vi "UPH & Target & Clear Zero.vi"(8 "error in (no error)":errorcluster, 11 "Main":T1={"Tite"="", "Base path"=path "", "Table"=[], "Stations"=[], "Shield Array"=[], "UPHs"=[], "VISA"={"VISA"="", "baud rate"=9600, "data bits"=8, "parity"=enum."None", "stop bits"=10, "flow control"=0}, "Path"={"roof"=path "", "Config"=path "", "Png"=path ""}, "Ctr"={"DB Dispaly"=refnum, "Error Table"=refnum, "Display"=refnum, "Login"=refnum, "Exit"=refnum, "FTT_Submit"=refnum}, "Login"={"User"="", "Grade"=""}, "information"={"cause"="", "Type"=enum."Inform", "code"=0, "Suroce"="", "Status"=FALSE}, "Local DB"={"Connstr"="", "Database"={"Constr"={"Driver"="", "Server"="", "User"="", "Pwd"="", "Database"=""}, "conn ref"=refnum, "State"=FALSE}}, "Remote DB"={"Connstr"="", "Database"={"Constr"={"Driver"="", "Server"="", "User"="", "Pwd"="", "Database"=""}, "conn ref"=refnum, "State"=FALSE}}, "FTT TV"="", "ExchangeTime"=0, "NVH"="", "EOL Path"=path ""} {"VISA"."flow control" items=["None", "XON/XOFF", "RTS/CTS", "XON/XOFF & RTS/CTS", "DTR/DSR", "XON/XOFF & DTR/DSR"]; "VISA"."stop bits" items=["1.0"=10, "1.5"=15, "2.0"=20]}) -> (0 "error out":errorcluster)   [LabVIEW 2014]
uses:
  <vilib>/addons/database/Connection.llb/Conn ObjectReference.ctl
  <vilib>/addons/database/NI_Database_API.lvlib
  Type'def/Online_Table.ctl
  Type'def/UPH Config.ctl
  <vilib>/ptbypt/NI_PtbyPt.lvlib
  VISA/Ctr/VISA Ctr.ctl
  Type'def/Main Ctr Ref.ctl
  Type'def/User Login.ctl
  Database/Ctr/Constr.ctl
  Database/Ctr/Conneect State.ctl
  Type'def/MainCtr.ctl
panel:
  in  "Boolean":bool
  out "Previous Event":string
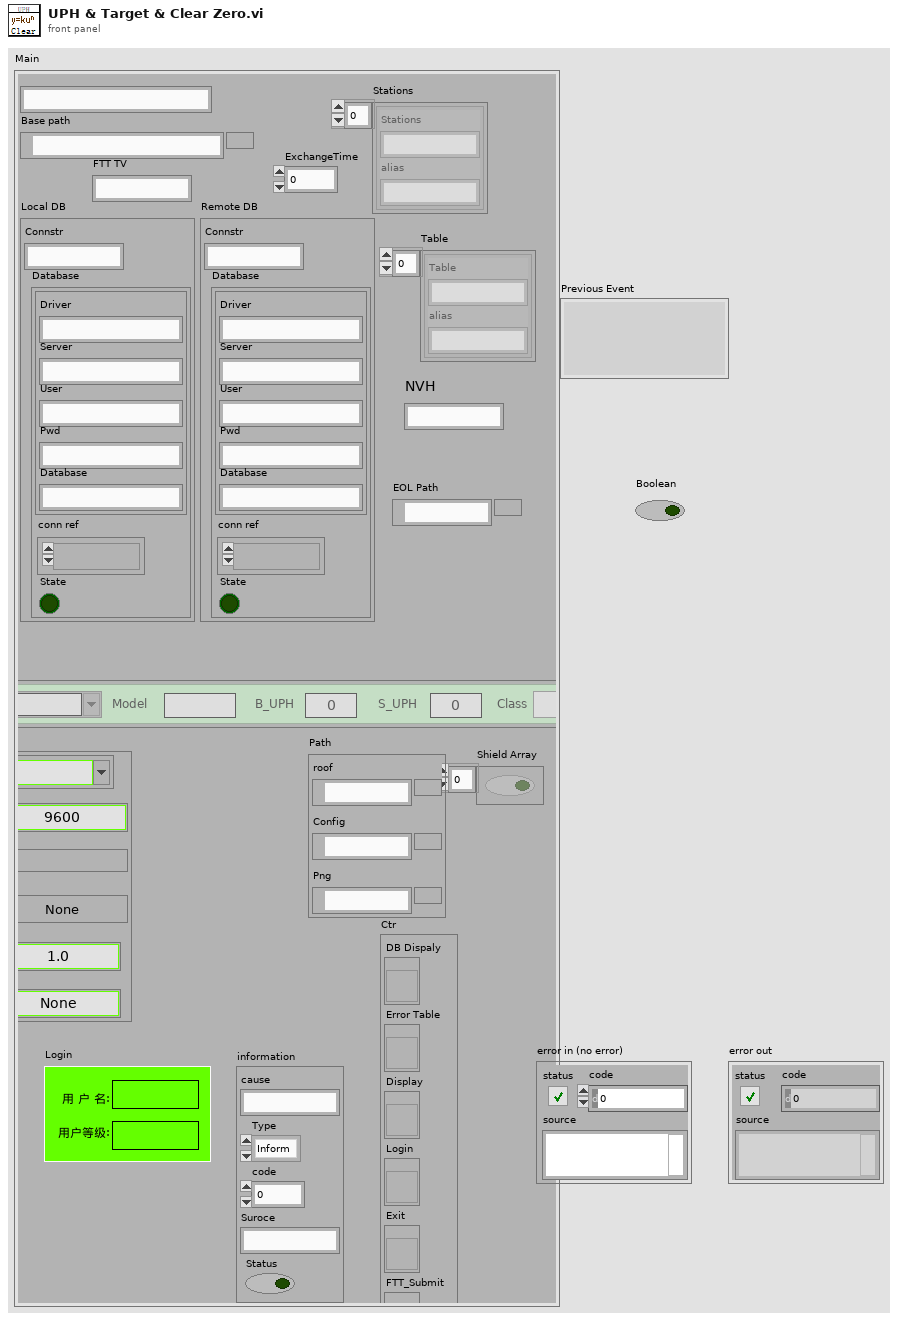
[diagram p1: front panel]
types:
  T1 = typedef "MainCtr.ctl" = cluster{"Tite":string, "Base path":path, "Table":cluster{"Table":string, "alias":string}[], "Stations":cluster{"Stations":string, "alias":string}[], "Shield Array":bool[], "UPHs":T2[], "VISA":T3, "Path":cluster{"roof":path, "Config":path, "Png":path}, "Ctr":T4, "Login":T5, "information":cluster{"cause":string, "Type":enum16{"Inform", "Warning", "Alarm"}, "code":i32, "Suroce":string, "Status":bool}, "Local DB":cluster{"Connstr":string, "Database":T6}, "Remote DB":cluster{"Connstr":string, "Database":T6}, "FTT TV":string, "ExchangeTime":i32, "NVH":string, "EOL Path":path}
  T2 = typedef "UPH Config.ctl" = cluster{"Line_No":string, "Model":string, "B_UPH ":i16, "S_UPH  ":i16, "Class":enum16{"Big", "Small"}}
  T3 = typedef "VISA Ctr.ctl" = cluster{"VISA":refnum<visa-resource-name>, "baud rate":u32, "data bits":u16, "parity":enum16{"None", "Odd", "Even", "Mark", "Space"}, "stop bits":u16, "flow control":u16}
  T4 = typedef "Main Ctr Ref.ctl" = cluster{"DB Dispaly":refnum<vi>, "Error Table":refnum<vi>, "Display":refnum<vi>, "Login":refnum<vi>, "Exit":refnum<vi>, "FTT_Submit":refnum<vi>}
  T5 = typedef "User Login.ctl" = cluster{"User":string, "Grade":string}
  T6 = typedef "Conneect State.ctl" = cluster{"Constr":T7, "conn ref":T8, "State":bool}
  T7 = typedef "Constr.ctl" = cluster{"Driver":string, "Server":string, "User":string, "Pwd":string, "Database":string}
  T8 = typedef "NI_Database_API.lvlib/Conn ObjectReference.ctl" = refnum<k1>
  T9 = typedef "Online_Table.ctl" = cluster{"SN":string, "Frame":string, "Station":string, "Model":string, "Color":string, "OnTime":timestamp, "OutTime":timestamp, "Repaired":i32, "OnRepair":bool, "Pstate":string}
  T10 = cluster{"cause":string, "Type":enum16{"Inform", "Warning", "Alarm"}, "code":i32, "Suroce":string, "Status":bool}
  T11 = cluster{"No Plan(s)":dbl, "Seconds":dbl, "Main ":T1, "Online_Table":T9, "information":cluster{"cause":string, "Type":enum16{"Inform", "Warning", "Alarm"}, "code":i32, "Suroce":string, "Status":bool}, "n":dbl, "uph":T2[]}
  T12 = typedef "FTT Display Type.ctl" = cluster{"Line.No":string, "Model":string, "Color":string, "UPH":dbl, "Plan":dbl, "Target Rate":dbl, "Target ":dbl, "Actual":dbl, "FTT":dbl, "FTT Rate":dbl, "Repaired":dbl, "Reject":dbl, "Ouline":dbl, "Line State":string}
  T13 = cluster{"Display":T12, "Class":enum16{"Big", "Small"}}
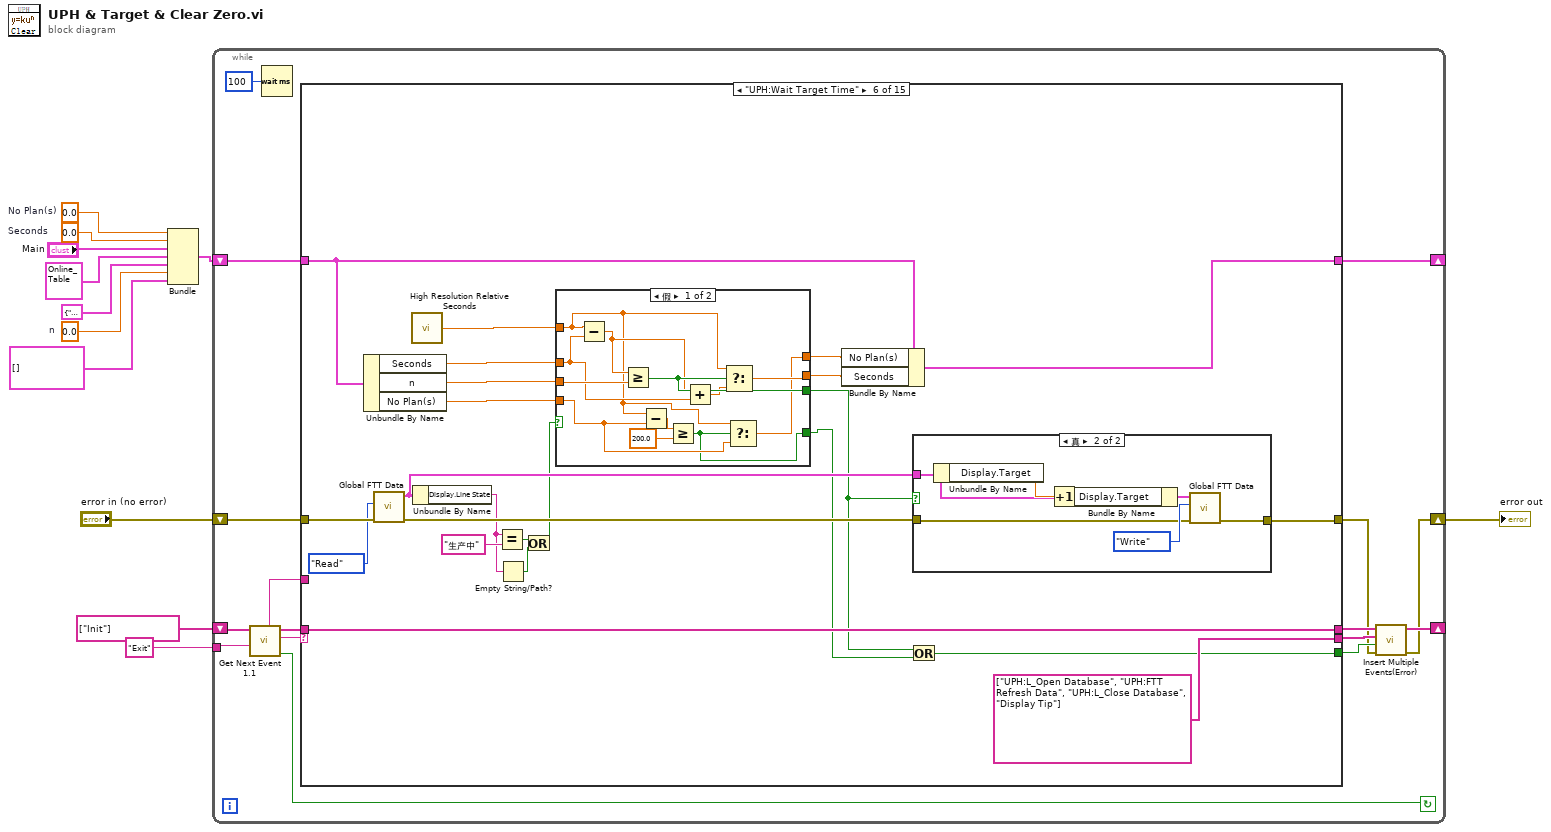
[diagram p0: block diagram]
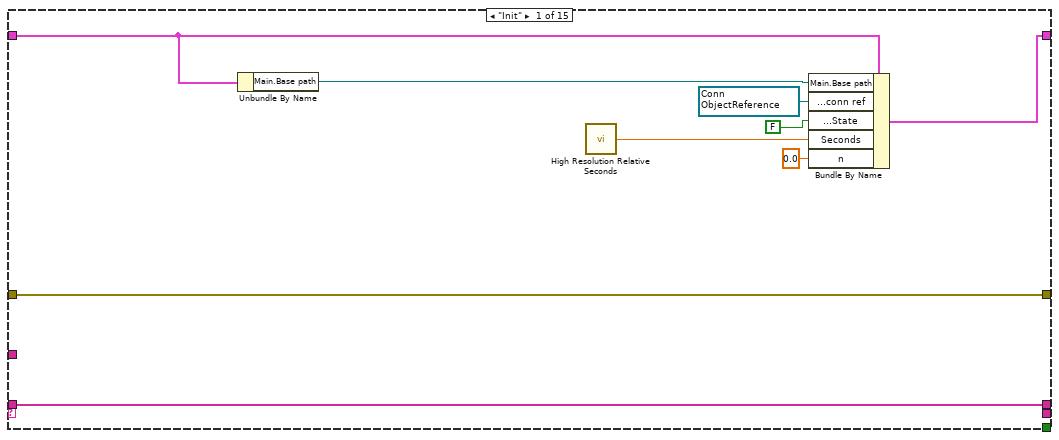
[diagram p2: hidden frame]
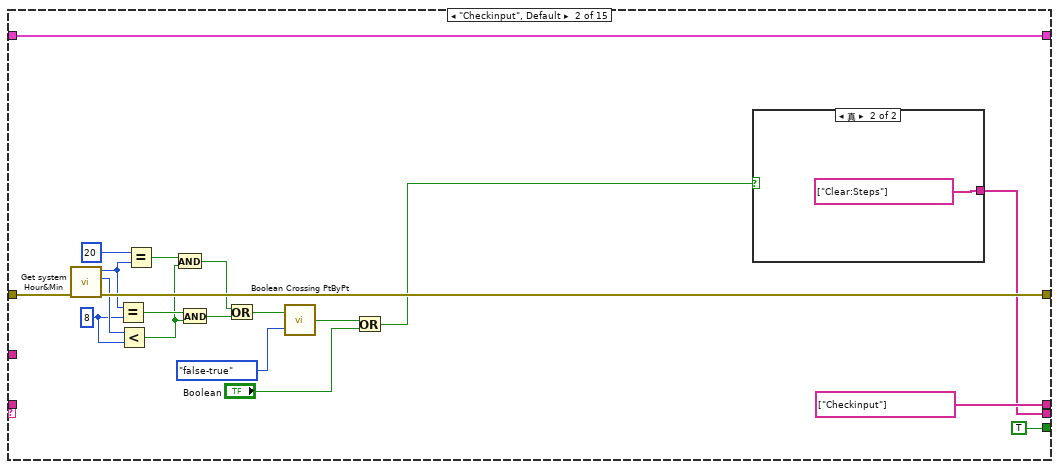
[diagram p3: hidden frame]
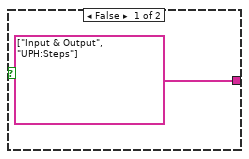
[diagram p4: hidden frame]
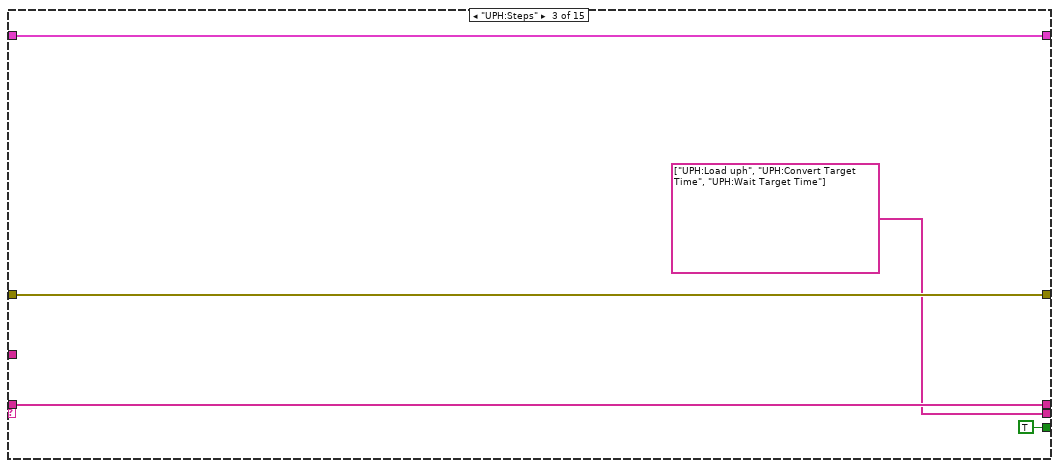
[diagram p5: hidden frame]
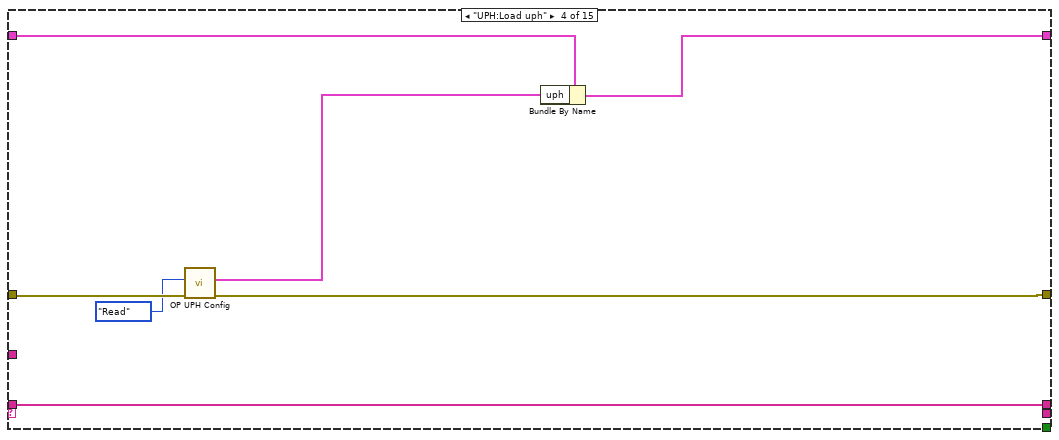
[diagram p6: hidden frame]
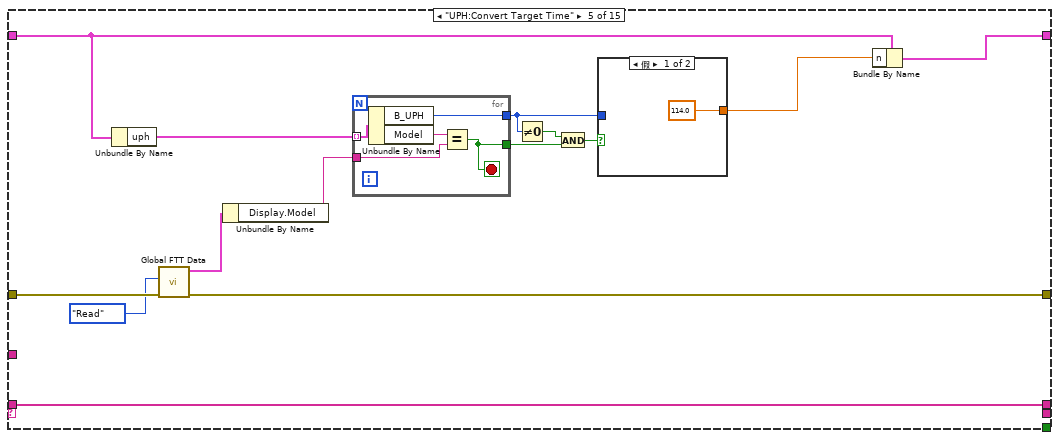
[diagram p7: hidden frame]
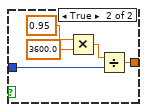
[diagram p8: hidden frame]
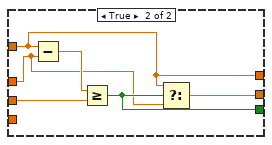
[diagram p10: hidden frame]
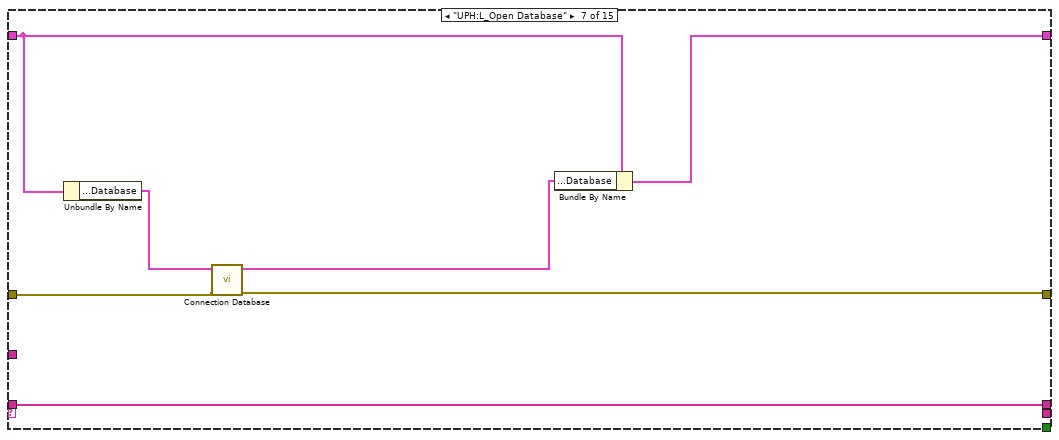
[diagram p11: hidden frame]
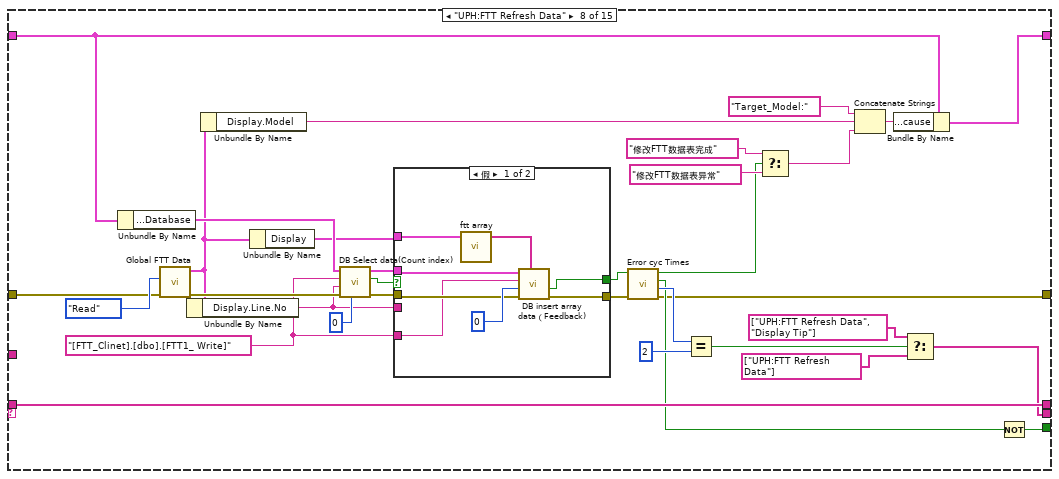
[diagram p12: hidden frame]
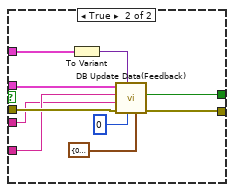
[diagram p13: hidden frame]
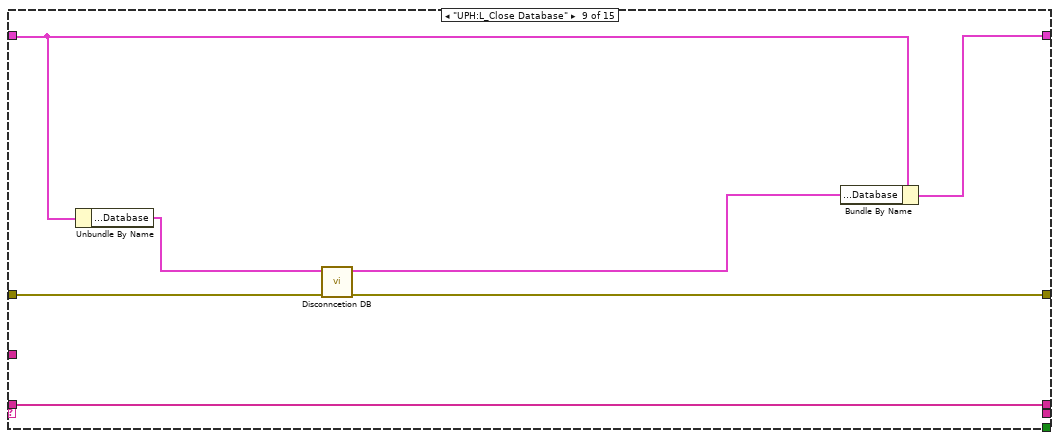
[diagram p14: hidden frame]
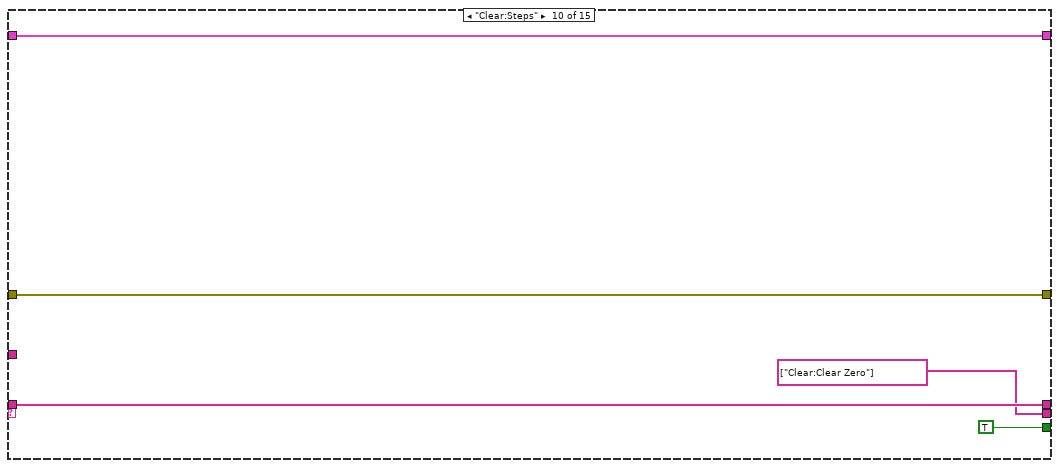
[diagram p15: hidden frame]
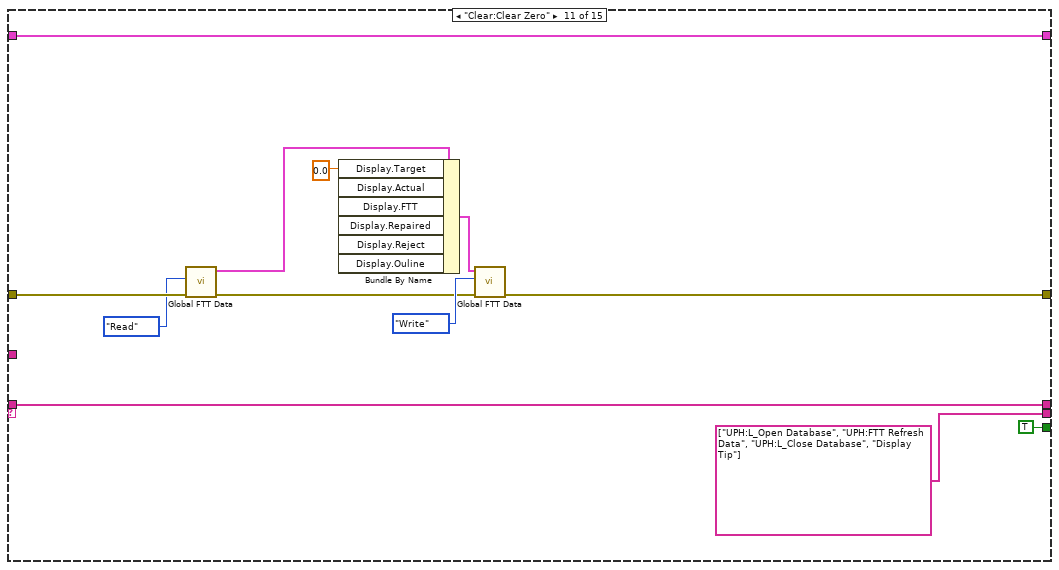
[diagram p16: hidden frame]
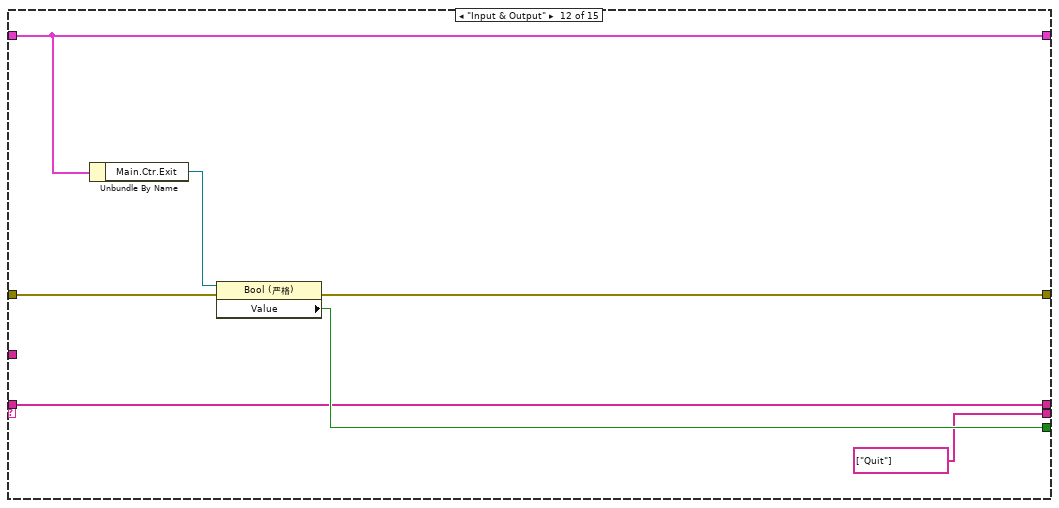
[diagram p17: hidden frame]
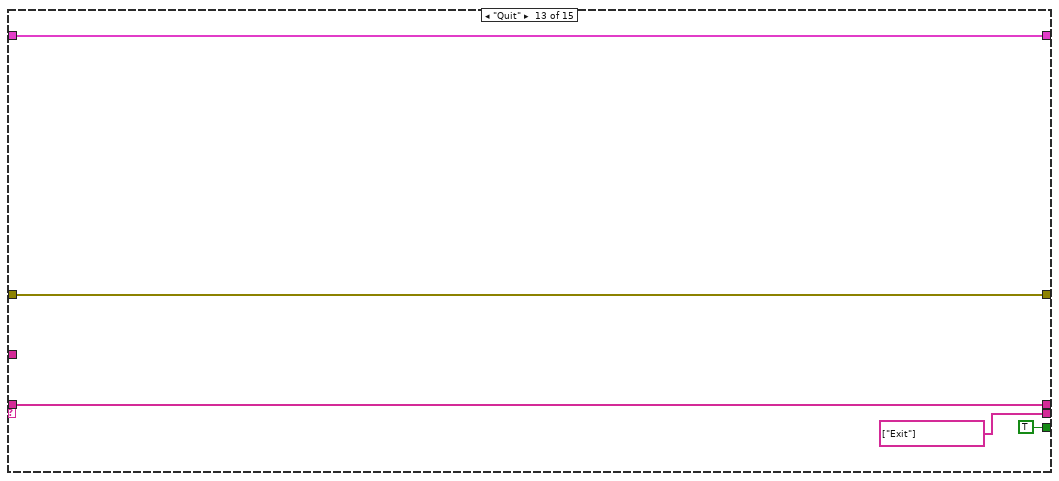
[diagram p18: hidden frame]
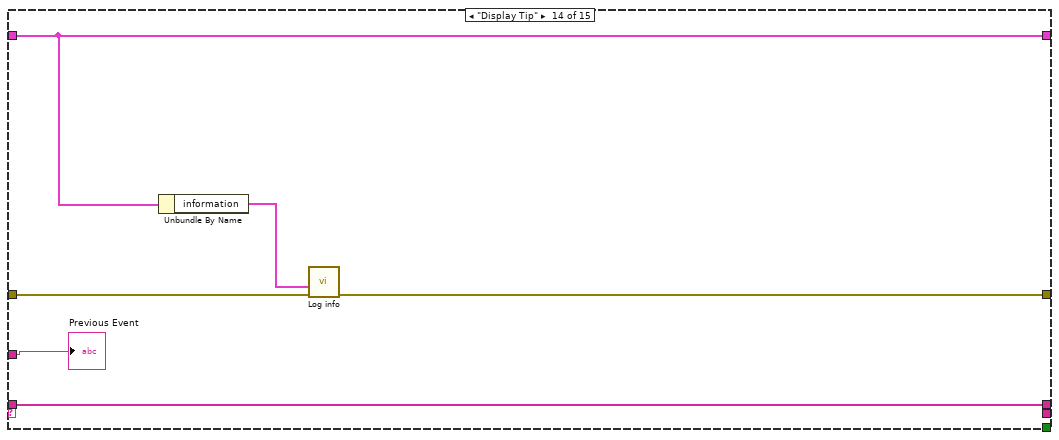
[diagram p19: hidden frame]
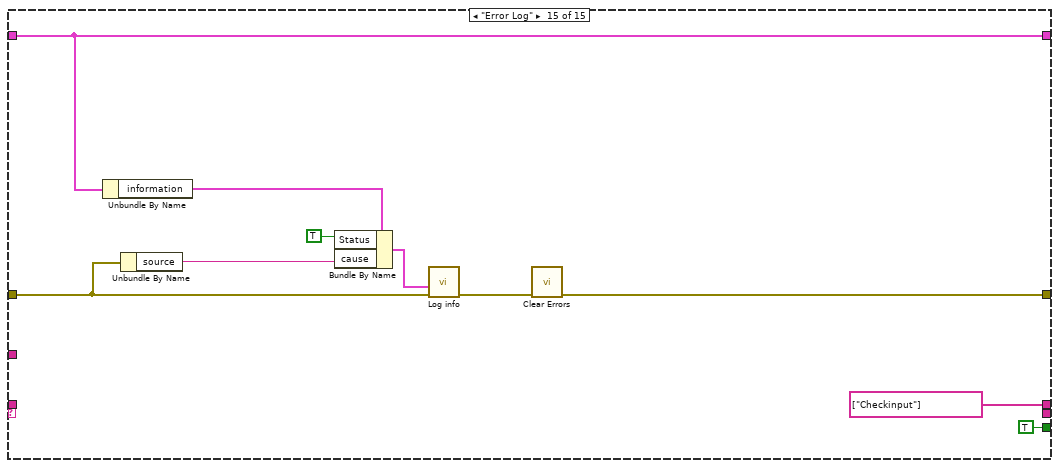
[diagram p20: hidden frame]
diagram:
  w1 = 0.0  # No Plan(s)
  w2 = 0.0  # Seconds
  w4 = 0.0  # n
  n1 = Bundle("No Plan(s)"=w1, "Seconds"=w2, "Main"="Main", "Online_Table"=T9 {"SN"="", "Frame"="", "Station"="", "Model"="", "Color"="", "OnTime"=timestamp(0 s since 1904-01-01), "OutTime"=timestamp(0 s since 1904-01-01), "Repaired"=0, "OnRepair"=FALSE, "Pstate"=""}, "information"=T10 {"cause"="", "Type"=enum."Inform", "code"=0, "Suroce"="", "Status"=FALSE}, "n"=w4, "uph"=T2[] []) -> (w9:T11)  [unwired: 1 in]
  n2 = while {
    tunnel: "Exit" ("Exit Event") -> [w25]
    shift-right: [w21] -> _
    shift-left: string[] ["Init"] -> [w26]
    shift-right: [w15] -> w6
    shift-left: "error in (no error)" -> [w24]
    shift-right: [w17] -> _
    shift-left: w9 -> [w22]
    stop <- w27 continue-if-true
    n3 = call "Get Next Event 1.1.vi"("Exit Event"=w25, "event queue in"=w26) -> ("Condition (Exit:F)"=w27:bool, "next event"=w28:string, "event queue out"=w23:string[], "Previous Event"=w13:string)  [unwired: 6 in]
    n4 = Wait (ms)(milliseconds to wait=u32 100) -> ()  [unwired: 1 out]
    n5 = case shown="\"UPH:Wait Target Time\"" w28 {
      tunnel: w24 -> [w36 w54 w63 w71 w85 w116 w152 w183 w210 w214 w225 w233 w238 w245 w248]
      tunnel: w23 -> [w37 _ w62 w65 w72 w119 w147 w177 w205 w213 w226 w229 w237 w241 _]
      tunnel: w22 -> [w34 w55 w64 w68 w75 w118 w150 w164 w208 w215 w227 w234 w239 w243 w253]
      tunnel: [w36 w53 w63 w69 w83 w108 w148 w162 w206 w214 w220 w231 w238 w244 w254] -> w16
      tunnel: [w37 string[] ["Checkinput"] w62 w65 w72 w119 w147 w177 w205 w213 w226 w229 w237 w241 string[] ["Checkinput"]] -> w20
      tunnel: [_ TRUE ("Insert all? (T)") TRUE ("Insert all? (T)") _ _ w98 _ w167 _ TRUE ("Insert all? (T)") TRUE ("Insert all? (T)") w230 TRUE ("Insert all? (T)") _ TRUE ("Insert all? (T)")] -> w19
      tunnel: [_ w45 string[] ["UPH:Load uph", "UPH:Convert Target Time", "UPH:Wait Target Time"] _ _ string[] ["UPH:L_Open Database", "UPH:FTT Refresh Data", "UPH:L_Close Database", "Display Tip"] _ w161 _ string[] ["Clear:Clear Zero"] string[] ["UPH:L_Open Database", "UPH:FTT Refresh Data", "UPH:L_Close Database", "Display Tip"] string[] ["Quit"] string[] ["Exit"] _ _] -> w18
      tunnel: [w35 w55 w64 w66 w74 w117 w146 w163 w204 w215 w227 w234 w239 w243 w253] -> w17
      tunnel: w13 -> [_ _ _ _ _ _ _ _ _ _ _ _ _ w240 _]
      frame "Init" {
        w32 = T8 refnum items=["Connection"] ("conn refer.conn ref")
        n6 = Unbundle By Name(w34) -> ("Main.Base path"=w33:path)
        n7 = call <vilib>:"High Resolution Relative Seconds.vi"() -> ("relative seconds"=w30:dbl)
        n8 = Bundle By Name(cluster=w34, "Main.Base path"=w33, "Main.Local DB.Database.conn ref"=w32, "Main.Local DB.Database.State"=FALSE ("conn refer.State"), "Seconds"=w30, "n"=0.0) -> (w35:T11)
      }
      frame "Checkinput", Default {
        w51 = 8
        n9 = call "Get system Hour&Min.vi"("error in (no error)"=w54) -> ("error out"=w53:errorcluster, "minute"=w52:i32, "hour"=w44:i32)  [unwired: 7 in, 1 out]
        n10 = Equal?(x=w44, y=w51) -> (x = y?=w50:bool)
        n11 = Less?(x=w52, y=w51) -> (x < y?=w41:bool)
        n12 = Equal?(x=20, y=w44) -> (x = y?=w42:bool)
        n13 = And(x=w42, y=w41) -> (x .and. y?=w39:bool)
        n14 = And(x=w50, y=w41) -> (x .and. y?=w40:bool)
        n15 = Or(x=w39, y=w40) -> (x .or. y?=w38:bool)
        n16 = call <vilib>:"Boolean Crossing PtByPt.vi"("direction"=enum16{"either", "false-true", "true-false"}."false-true", "input"=w38) -> ("crossing"=w48:bool)  [unwired: 1 in]
        n17 = Or(x=w48, y="Boolean") -> (x .or. y?=w46:bool)
        n18 = case shown="真" w46 {
          tunnel: [string[] ["Input & Output", "UPH:Steps"] string[] ["Clear:Steps"]] -> w45
          frame False {
          }
          frame True {
          }
        }
      }
      frame "UPH:Steps" {
      }
      frame "UPH:Load uph" {
        n19 = call "OP UPH Config.vi"("error in (no error)"=w71, "Enum"=enum16{"init", "Read", "Write"}."Read") -> ("error out"=w69:errorcluster, "UPH out"=w67:T2[])  [unwired: 7 in, 1 out]
        n20 = Bundle By Name(cluster=w68, "uph"=w67) -> (w66:T11)
      }
      frame "UPH:Convert Target Time" {
        n21 = Unbundle By Name(w75) -> ("uph"=w81:T2[])
        n22 = call "Global FTT Data.vi"("error in (no error)"=w85, "Mode"=enum16{"Read", "Write"}."Read") -> ("error out"=w83:errorcluster, "Cluster"=w82:T13)  [unwired: 8 in]
        n23 = Unbundle By Name(w82) -> ("Display.Model"=w80:string)
        n24 = for {
          tunnel: w81 -> [w96] mode=indexing
          tunnel: w80 -> [w94]
          tunnel: [w93] -> w76
          tunnel: [w92] -> w79
          stop <- w92 stop-if-true
          n25 = Unbundle By Name(w96) -> ("B_UPH"=w93:i16, "Model"=w95:string)
          n26 = Equal?(x=w95, y=w94) -> (x = y?=w92:bool)
        }
        n27 = Not Equal To 0?(x=w76) -> (x != 0?=w78:bool)
        n28 = And(x=w78, y=w79) -> (x .and. y?=w77:bool)
        n29 = case shown="假" w77 {
          tunnel: w76 -> [_ w88]
          tunnel: [114.0 w87] -> w73
          frame False {
          }
          frame True {
            n30 = Multiply(x=0.95, y=3600.0) -> (x*y=w89:dbl)
            n31 = Divide(x=w89, y=w88) -> (x/y=w87:dbl)
          }
        }
        n32 = Bundle By Name(cluster=w75, "n"=w73) -> (w74:T11)
      }
      frame "UPH:Wait Target Time" {
        n33 = Unbundle By Name(w118) -> ("Seconds"=w115:dbl, "n"=w113:dbl, "No Plan(s)"=w100:dbl)
        n34 = call "Global FTT Data.vi"("error in (no error)"=w116, "Mode"=enum16{"Read", "Write"}."Read") -> ("error out"=w109:errorcluster, "Cluster"=w110:T13)  [unwired: 8 in]
        n35 = call <vilib>:"High Resolution Relative Seconds.vi"() -> ("relative seconds"=w114:dbl)
        n36 = Unbundle By Name(w110) -> ("Display.Line State"=w105:string)
        n37 = Equal?(x=w105, y="生产中") -> (x = y?=w103:bool)
        n38 = Empty String/Path?(string/path=w105) -> (empty?=w104:bool)
        n39 = Or(x=w103, y=w104) -> (x .or. y?=w102:bool)
        n40 = case shown="假" w102 {
          tunnel: w115 -> [w135 w141]
          tunnel: w114 -> [w129 w140]
          tunnel: w113 -> [w139 w143]
          tunnel: [w138 w142] -> w99
          tunnel: [w134 w144] -> w112
          tunnel: [w131 w140] -> w101
          tunnel: w100 -> [w130 _]
          tunnel: [w128 _] -> w97
          frame False {
            n41 = Subtract(x=w129, y=w135) -> (x-y=w136:dbl)
            n42 = Greater Or Equal?(x=w136, y=w139) -> (x >= y?=w138:bool)
            n43 = Subtract(x=w129, y=w130) -> (x-y=w133:dbl)
            n44 = Greater Or Equal?(x=w133, y=200.0) -> (x >= y?=w128:bool)
            n45 = Add(x=w136, y=w135) -> (x+y=w137:dbl)
            n46 = Select(t=w129, s=w138, f=w137) -> (s? t:f=w134:dbl)
            n47 = Select(t=w129, s=w128, f=w130) -> (s? t:f=w131:dbl)
          }
          frame True {
            n48 = Subtract(x=w140, y=w141) -> (x-y=w145:dbl)
            n49 = Greater Or Equal?(x=w145, y=w143) -> (x >= y?=w142:bool)
            n50 = Select(t=w140, s=w142, f=w141) -> (s? t:f=w144:dbl)
          }
        }
        n51 = Bundle By Name(cluster=w118, "No Plan(s)"=w101, "Seconds"=w112) -> (w117:T11)
        n52 = Or(x=w99, y=w97) -> (x .or. y?=w98:bool)
        n53 = case shown="真" w99 {
          tunnel: w110 -> [_ w122]
          tunnel: w109 -> [w120 w124]
          tunnel: [w120 w121] -> w108
          frame False {
          }
          frame True {
            n54 = Unbundle By Name(w122) -> ("Display.Target"=w123:dbl)
            n55 = Increment(x=w123) -> (x+1=w127:dbl)
            n56 = Bundle By Name(cluster=w122, "Display.Target"=w127) -> (w126:T13)
            n57 = call "Global FTT Data.vi"("error in (no error)"=w124, "Mode"=enum16{"Read", "Write"}."Write", "Display"=w126) -> ("error out"=w121:errorcluster)  [unwired: 7 in, 1 out]
          }
        }
      }
      frame "UPH:L_Open Database" {
        n58 = Unbundle By Name(w150) -> ("Main.Local DB.Database"=w151:T6)
        n59 = call "Connection Database.vi"("error in (no error)"=w152, "Connncet State"=w151) -> ("error out"=w148:errorcluster, "Connncet State out"=w149:T6)  [unwired: 8 in]
        n60 = Bundle By Name(cluster=w150, "Main.Local DB.Database"=w149) -> (w146:T11)
      }
      frame "UPH:FTT Refresh Data" {
        w155 = "[FTT_Clinet].[dbo].[FTT1_ Write]"
        n61 = Unbundle By Name(w164) -> ("Main.Local DB.Database"=w185:T6)
        n62 = call "Global FTT Data.vi"("error in (no error)"=w183, "Mode"=enum16{"Read", "Write"}."Read") -> ("error out"=w182:errorcluster, "Cluster"=w154:T13)  [unwired: 8 in]
        n63 = Unbundle By Name(w154) -> ("Display.Line.No"=w176:string)
        n64 = Unbundle By Name(w154) -> ("Display.Model"=w160:string)
        n65 = Unbundle By Name(w154) -> ("Display"=w153:T12)
        n66 = call "DB Select data(Count index).vi"("index"=0, "error in (no error)"=w182, "Code"=w176, "Tabe"=w155, "Connncet State"=w185) -> ("error out"=w180:errorcluster, "state"=w179:bool, "Connncet State out"=w178:T6)  [unwired: 3 in, 1 out]
        n67 = case shown="假" w179 {
          tunnel: w180 -> [w191 w201]
          tunnel: w178 -> [w190 w200]
          tunnel: w153 -> [w189 w195]
          tunnel: w155 -> [w188 w199]
          tunnel: [w187 w197] -> w169
          tunnel: w176 -> [_ w198]
          tunnel: [w186 w196] -> w168
          frame False {
            n68 = call "ftt array.vi"("Display"=w189) -> ("appended array"=w192:string[])  [unwired: 4 in]
            n69 = call "DB insert array data（Feedback).vi"("Data"=w192, "error in (no error)"=w191, "index"=0, "table"=w188, "Connncet State"=w190) -> ("error out"=w187:errorcluster, "state"=w186:bool)  [unwired: 4 in, 1 out]
          }
          frame True {
            n70 = To Variant(anything=w195) -> (Variant=w194:variant)
            n71 = call "DB Update Data(Feedback).vi"("Pos"=cluster{"index":i32, "Len":i32} {"index"=0, "Len"=14}, "Sel index"=0, "data"=w194, "error in (no error)"=w201, "Code"=w198, "table"=w199, "Connncet State"=w200) -> ("error out"=w197:errorcluster, "State"=w196:bool)  [unwired: 2 in, 1 out]
          }
        }
        n72 = call "Error cyc Times.vi"("error in (no error)"=w169, "Status in"=w168) -> ("error out"=w162:errorcluster, "Numeric"=w170:i32, "Cys Status"=w166:bool, "Status out"=w157:bool)  [unwired: 6 in]
        n73 = Equal?(x=w170, y=2) -> (x = y?=w172:bool)
        n74 = Select(t="修改FTT数据表完成", s=w157, f="修改FTT数据表异常") -> (s? t:f=w158:string)
        n75 = Concatenate Strings("Target_Model:" ("information.cause"), w160, w158) -> (w165:string)
        n76 = Bundle By Name(cluster=w164, "information.cause"=w165) -> (w163:T11)
        n77 = Select(t=string[] ["UPH:FTT Refresh Data", "Display Tip"], s=w172, f=string[] ["UPH:FTT Refresh Data"]) -> (s? t:f=w161:string[])
        n78 = Not(x=w166) -> (.not. x?=w167:bool)
      }
      frame "UPH:L_Close Database" {
        n79 = Unbundle By Name(w208) -> ("Main.Local DB.Database"=w209:T6)
        n80 = call "Disconncetion DB.vi"("error in (no error)"=w210, "Connncet State"=w209) -> ("error out"=w206:errorcluster, "Connect State"=w207:T6)  [unwired: 8 in]
        n81 = Bundle By Name(cluster=w208, "Main.Local DB.Database"=w207) -> (w204:T11)
      }
      frame "Clear:Steps" {
      }
      frame "Clear:Clear Zero" {
        w218 = 0.0
        n82 = call "Global FTT Data.vi"("error in (no error)"=w225, "Mode"=enum16{"Read", "Write"}."Read") -> ("error out"=w221:errorcluster, "Cluster"=w223:T13)  [unwired: 8 in]
        n83 = Bundle By Name(cluster=w223, "Display.Target"=w218, "Display.Actual"=w218, "Display.FTT"=w218, "Display.Repaired"=w218, "Display.Reject"=w218, "Display.Ouline"=w218) -> (w219:T13)
        n84 = call "Global FTT Data.vi"("error in (no error)"=w221, "Mode"=enum16{"Read", "Write"}."Write", "Display"=w219) -> ("error out"=w220:errorcluster)  [unwired: 7 in, 1 out]
      }
      frame "Input & Output" {
        n85 = Unbundle By Name(w234) -> ("Main.Ctr.Exit"=w232:refnum<vi>)
        n86 = property class="Bool (严格)"(reference=w232, error in=w233) -> (error out=w231:errorcluster, "Value"=w230:bool)  [unwired: 1 out]
      }
      frame "Quit" {
      }
      frame "Display Tip" {
        n87 = Unbundle By Name(w243) -> ("information"=w242:T10)
        n88 = call "Log info.vi"("error in (no error)"=w245, "information"=w242) -> ("error out"=w244:errorcluster)  [unwired: 8 in, 1 out]
        "Previous Event" <- w240
      }
      frame "Error Log" {
        n89 = Unbundle By Name(w253) -> ("information"=w252:T10)
        n90 = Unbundle By Name(w248) -> ("source"=w247:string)
        n91 = Bundle By Name(cluster=w252, "Status"=TRUE, "cause"=w247) -> (w251:T10)
        n92 = call "Log info.vi"("error in (no error)"=w248, "information"=w251) -> ("error out"=w255:errorcluster)  [unwired: 8 in, 1 out]
        n93 = call <vilib>:"Clear Errors.vi"("error in (no error)"=w255) -> ("error out"=w254:errorcluster)  [unwired: 5 in, 1 out]
      }
    }
    n94 = call "Insert Multiple Events(Error).vi"("error in (no error)"=w16, "Insert all? (T)"=w19, "Events to Insert"=w18, "Event queue in"=w20) -> ("error out"=w15:errorcluster, "Event queue out"=w21:string[])  [unwired: 6 in]
  }
  "error out" <- w6
